vi "Move Linked List.vi"(6 "Insertion Index":i32=-1, 7 "New Parent Linked List ID":string, 8 "error in (no error)":errorcluster, 10 "Linked List ID":string, 11 "Linked List in":refnum<class "Linked List.lvclass">) -> (0 "error out":errorcluster, 2 "Linked List ID out":string, 3 "Linked List out":refnum<class "Linked List.lvclass">)   [LabVIEW 2020, in "Linked Lists.lvlib" / "Linked List.lvclass"]
uses:
  <vilib>/gpm_packages/@cs/linked-list/Source/Linked List/Linked List/Linked List.lvclass
  <vilib>/gpm_packages/@cs/linked-list/Source/Linked List/Linked List Definition/Linked List Definition.lvclass
  <vilib>/gpm_packages/@cs/linked-list/Source/Linked List/Linked List/Linked List.lvclass/Linked List.ctl
  <vilib>/gpm_packages/@cs/lookup-table/Source/LookupTable/LookupTable.lvclass/LookupTable.ctl
  dea0f38d-61f3-466e-aa12-9ceaa26f2994.vi
  <vilib>/gpm_packages/@cs/lookup-table/Source/LookupTable/Read Table Reference.vi
  dea0f38d-61f3-466e-aa12-9ceaa26f2994.vi/5a7267ad-595e-4610-9ac2-8bef780848ff.vi
  <vilib>/gpm_packages/@cs/lookup-table/Source/LookupTable/LookupTable.lvclass
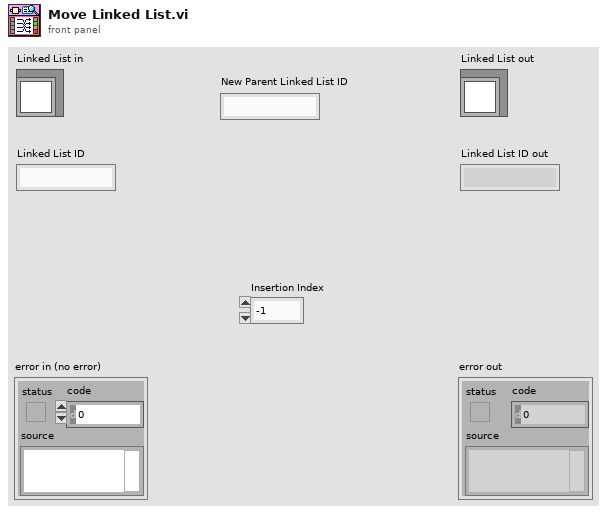
[diagram p1: front panel]
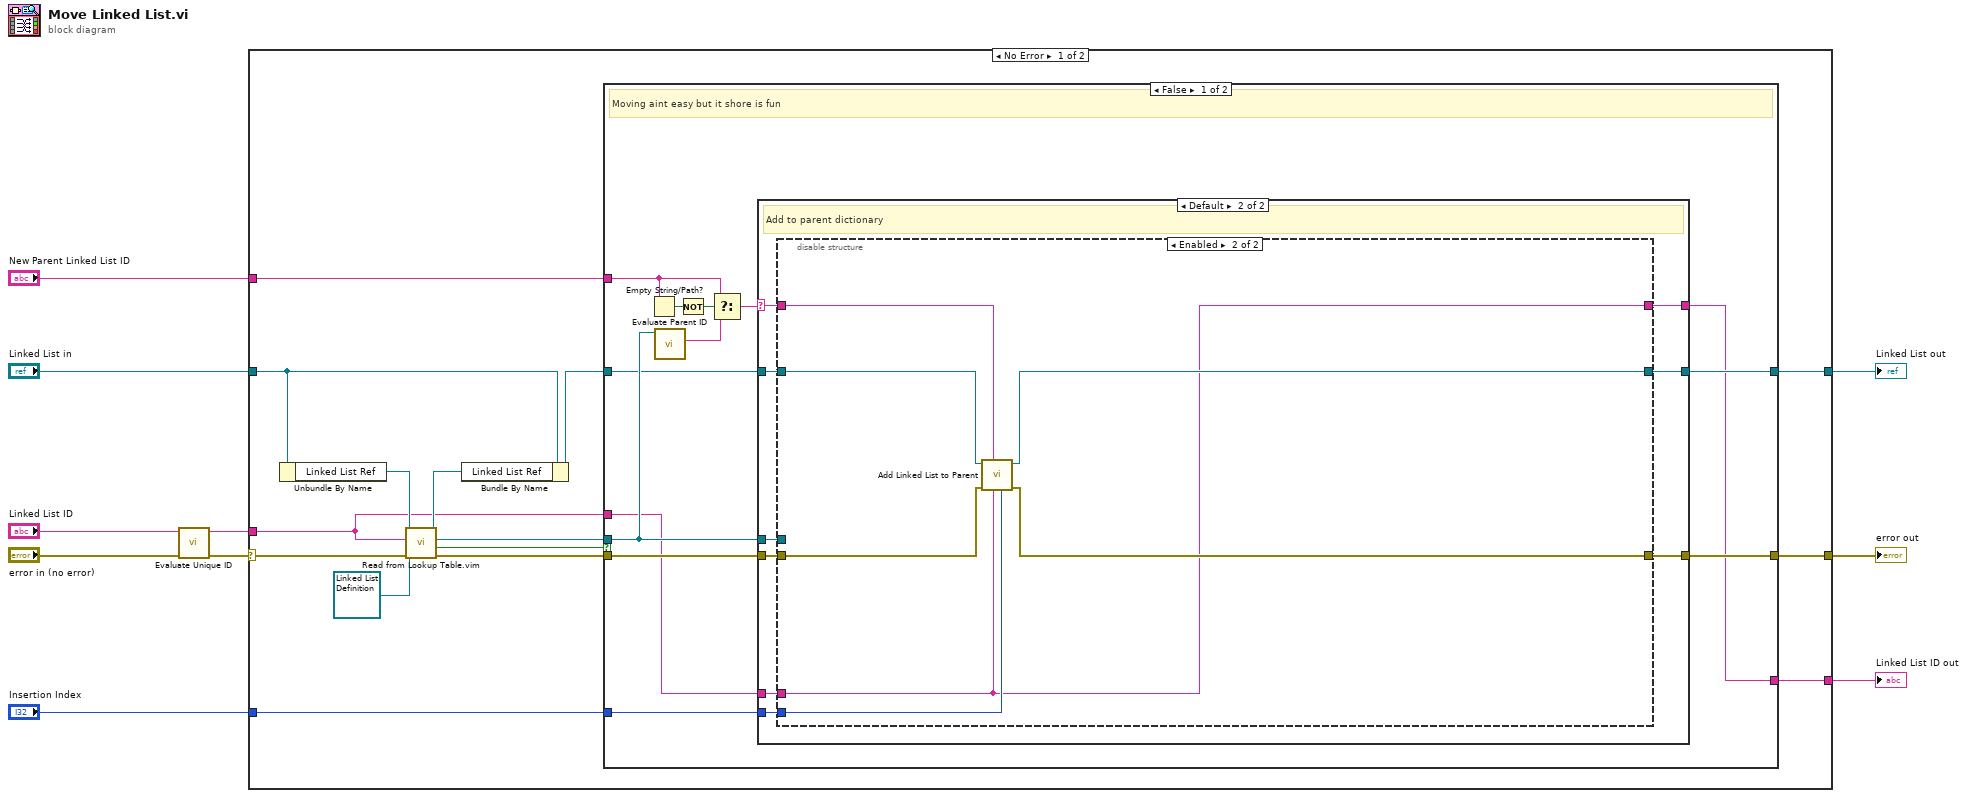
[diagram p0: block diagram]
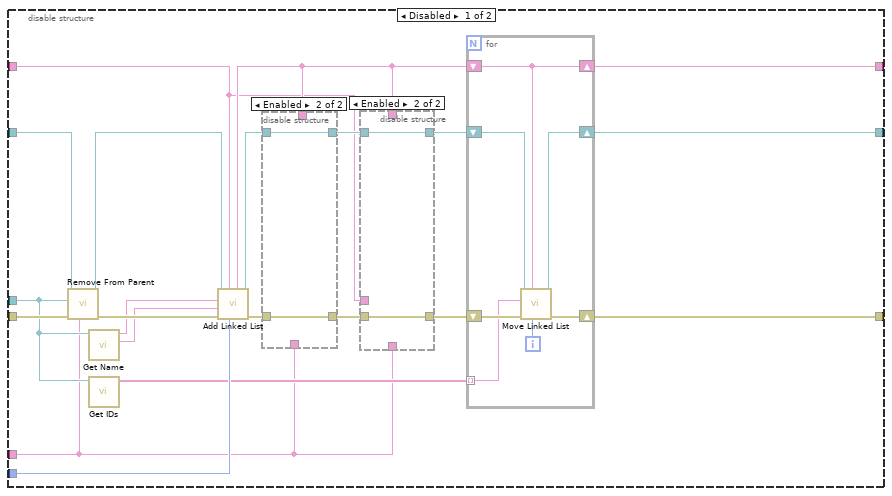
[diagram p3: hidden frame]
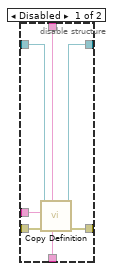
[diagram p4: hidden frame]
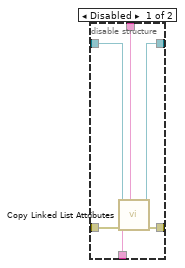
[diagram p5: hidden frame]
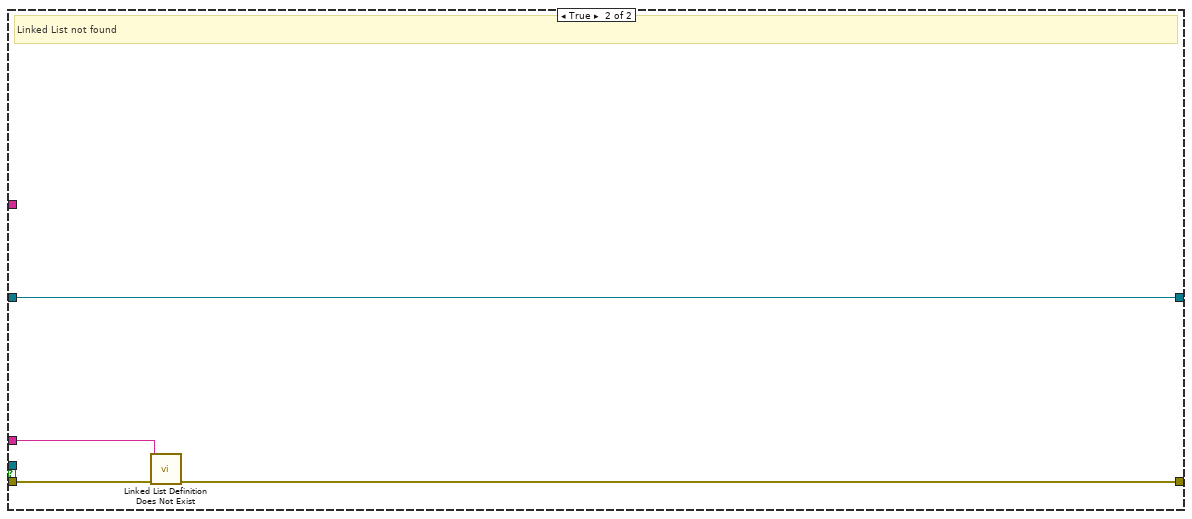
[diagram p6: hidden frame]
diagram:
  n1 = call <vilib>:"Evaluate Unique ID.vi"("error in (no error)"="error in (no error)", "Unique ID"="Linked List ID") -> ("error out"=w8:errorcluster, "Unique ID Out"=w7:string)  [unwired: 8 in]
  n2 = case shown="No Error" w8 {
    selector: w8 -> [w23 w107]
    tunnel: w7 -> [w11 _]
    tunnel: "Linked List in" -> [w18 w108]
    tunnel: [w16 w108] -> w5
    tunnel: [w15 w107] -> w4
    tunnel: "New Parent Linked List ID" -> [w14 _]
    tunnel: "Insertion Index" -> [w13 _]
    tunnel: [w12 _] -> w1
    frame No Error {
      n3 = Unbundle By Name(w18) -> ("Linked List Ref"=w25:refnum<data-value>)
      n4 = call "Read from Lookup Table.vim"("error in (no error)"=w23, "Type"=refnum<class "Linked List Definition.lvclass"> refnum ("Linked List.lvlib:Linked List Definition.lvclass"), "Item Name"=w11, "LookupTable Reference"=w25) -> ("error out"=w21:errorcluster, "Not Found?"=w22:bool, "Value"=w20:refnum<class "Linked List Definition.lvclass">, "LookupTable Reference Out"=w19:refnum<data-value>)  [unwired: 4 in]
      n5 = Bundle By Name(cluster=w18, "Linked List Ref"=w19) -> (w17:refnum<class "Linked List.lvclass">)
      n6 = case shown="False" w22 {
        tunnel: w21 -> [w34 w105]
        tunnel: w20 -> [w36 _]
        tunnel: w17 -> [w35 w106]
        tunnel: [w33 w106] -> w16
        tunnel: [w32 w104] -> w15
        tunnel: w14 -> [w38 _]
        tunnel: w13 -> [w37 _]
        tunnel: [w30 _] -> w12
        tunnel: w11 -> [w31 w103]
        frame False {
          # "Moving aint easy but it shore is fun"
          n7 = Empty String/Path?(string/path=w38) -> (empty?=w29:bool)
          n8 = call <vilib>:"Evaluate Parent ID.vi"("Linked List Definition in"=w36) -> ("Parent ID"=w27:string)  [unwired: 8 in, 2 out]
          n9 = Not(x=w29) -> (.not. x?=w28:bool)
          n10 = Select(t=w38, s=w28, f=w27) -> (s? t:f=w26:string)
          n11 = case shown="Default" w26 {
            selector: w26 -> [w39 w44]
            tunnel: w34 -> [w40 w49]
            tunnel: [w40 w42] -> w32
            tunnel: w35 -> [w41 w50]
            tunnel: [w41 w43] -> w33
            tunnel: w31 -> [_ w45]
            tunnel: w37 -> [_ w48]
            tunnel: [w39 w46] -> w30
            tunnel: w36 -> [_ w47]
            frame "" {
              # "No parent, should never execute"
            }
            frame Default {
              # "Add to parent dictionary"
              n12 = disable-structure shown="Enabled" {
                disable-tunnel: w50 -> [w71 w102]
                disable-tunnel: w49 -> [w70 w99]
                disable-tunnel: w48 -> [w67 w101]
                disable-tunnel: w47 -> [w63 _]
                disable-tunnel: [w61 w97] -> w46
                disable-tunnel: w45 -> [w55 w97]
                disable-tunnel: w44 -> [w54 w96]
                disable-tunnel: [w52 w100] -> w43
                disable-tunnel: [w51 w98] -> w42
                frame Disabled {
                  n13 = call <vilib>:"Remove From Parent.vi"("Unique ID"=w55, "error in (no error)"=w70, "Linked List Definition"=w63, "Linked List in"=w71) -> ("error out"=w69:errorcluster, "Linked List out"=w68:refnum<class "Linked List.lvclass">)  [unwired: 6 in]
                  n14 = call <vilib>:"Get Name.vi"("Linked List Definition in"=w63) -> ("Unique ID"=w53:string, "Name"=w66:string)  [unwired: 8 in, 1 out]
                  n15 = call <vilib>:"Get IDs.vi"("Linked List Definition in"=w63) -> ("Child IDs"=w62:string[])  [unwired: 8 in, 2 out]
                  n16 = call-dynamic "Add Linked List.vi"("Insertion Index"=w67, "Parent ID"=w54, "error in (no error)"=w69, "Unique ID"=w53, "Name"=w66, "Linked List in"=w68) -> ("error out"=w64:errorcluster, "Linked List out"=w65:refnum<class "Linked List.lvclass">, "Unique ID out"=w56:string)  [unwired: 2 in, 1 out]
                  n17 = disable-structure shown="Enabled" {
                    disable-tunnel: w65 -> [w86 w88]
                    disable-tunnel: w64 -> [w85 w87]
                    disable-tunnel: [w84 w87] -> w60
                    disable-tunnel: [w83 w88] -> w58
                    disable-tunnel: w56 -> [w82 _]
                    disable-tunnel: w55 -> [w81 _]
                    frame Disabled {
                      n18 = call-dynamic "Copy Linked List Attributes.vi"("Sink Linked List ID"=w82, "error in (no error)"=w85, "Source Linked List ID"=w81, "Linked List in"=w86) -> ("error out"=w84:errorcluster, "Linked List out"=w83:refnum<class "Linked List.lvclass">)  [unwired: 6 in]
                    }
                    frame Enabled {
                    }
                  }
                  n19 = disable-structure shown="Enabled" {
                    disable-tunnel: w60 -> [w78 w79]
                    disable-tunnel: [w77 w79] -> w59
                    disable-tunnel: w58 -> [w76 w80]
                    disable-tunnel: [w75 w80] -> w57
                    disable-tunnel: w56 -> [w74 _]
                    disable-tunnel: w55 -> [w73 _]
                    disable-tunnel: w54 -> [w72 _]
                    frame Disabled {
                      n20 = call-dynamic "Copy Definition.vi"("Source Linked List ID"=w73, "Sink Linked List ID"=w74, "error in (no error)"=w78, "Sink Parent Linked List ID"=w72, "Linked List in"=w76) -> ("error out"=w77:errorcluster, "Linked List out"=w75:refnum<class "Linked List.lvclass">)  [unwired: 5 in]
                    }
                    frame Enabled {
                    }
                  }
                  n21 = for {
                    shift-right: [w94] -> w51
                    shift-left: w59 -> [w95]
                    shift-right: [w92] -> w52
                    shift-left: w57 -> [w93]
                    tunnel: w62 -> [w91] mode=indexing
                    shift-right: [w90] -> w61
                    shift-left: w56 -> [w90]
                    i -> [w89]
                    n22 = call-dynamic "Move Linked List.vi"("Insertion Index"=w89, "New Parent Linked List ID"=w90, "error in (no error)"=w95, "Linked List ID"=w91, "Linked List in"=w93) -> ("error out"=w94:errorcluster, "Linked List out"=w92:refnum<class "Linked List.lvclass">)  [unwired: 4 in, 1 out]
                  }
                }
                frame Enabled {
                  n23 = call-dynamic "Add Linked List to Parent.vi"("Insertion Index"=w101, "Linked List ID"=w97, "Parent ID"=w96, "error in (no error)"=w99, "Linked List in"=w102) -> ("error out"=w98:errorcluster, "Linked List out"=w100:refnum<class "Linked List.lvclass">)  [unwired: 5 in]
                }
              }
            }
          }
        }
        frame True {
          # "Linked List not found"
          n24 = call <vilib>:"Linked List Definition Does Not Exist.vi"("Error In"=w105, "Unique ID"=w103) -> ("Error Out"=w104:errorcluster)  [unwired: 9 in]
        }
      }
    }
    frame Error {
    }
  }
  "error out" <- w4
  "Linked List out" <- w5
  "Linked List ID out" <- w1
